vi "Drive Sizes.vi"(8 "error in (no error)":errorcluster, 11 "Windows System SAL in":refnum<class "Windows System SAL.lvclass">) -> (0 "error out":errorcluster, 3 "Windows System SAL out":refnum<class "Windows System SAL.lvclass">)   [LabVIEW 2020, in "Volatus.lvlib" / "Windows System SAL.lvclass"]
uses:
  Windows System SAL.lvclass
  Windows System SAL.lvclass/Windows System SAL.ctl
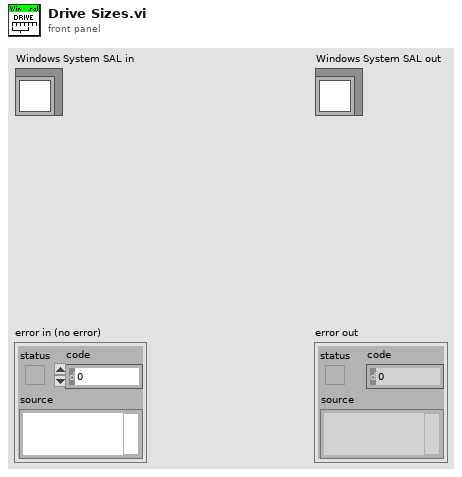
[diagram p1: front panel]
types:
  T1 = typedef "Volatus.lvlib/Windows System SAL.lvclass/Drive Info.ctl" = cluster{"Size GB":dbl, "Free GB":dbl}
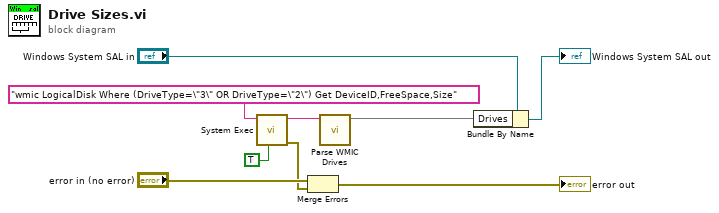
[diagram p0: block diagram]
diagram:
  n1 = call <vilib>:"System Exec.vi"("run minimized? (F)"=TRUE, "command line"="wmic LogicalDisk Where (DriveType=\"3\" OR DriveType=\"2\") Get DeviceID,FreeSpace,Size") -> ("error out"=w3:errorcluster, "standard output"=w6:string)  [unwired: 6 in, 2 out]
  n2 = Merge Errors("error in (no error)", w3) -> (→"error out":errorcluster)
  n3 = call "Parse WMIC Drives.vi"("WMIC Result"=w6) -> ("Drives"=w1:map{string, T1})  [unwired: 10 in]
  n4 = Bundle By Name(cluster="Windows System SAL in", "Drives"=w1) -> (→"Windows System SAL out":refnum<class "Windows System SAL.lvclass">)
